vi "auton_parse.vi"() -> ()   [LabVIEW 2015]
doc: "This VI is called when autonomous begins, and will automatically be terminated when autonomous ends. You can carry out timed or sensor driven robot movement independently without needing to return to the caller."
uses:
  auto_data.vi
panel:
  in  "auton_names":string[](array[string])=["none.bee", "", "", "", "", ""]
  # "Read a list of files from the filesystem\nParse them all into a giant command vector array"
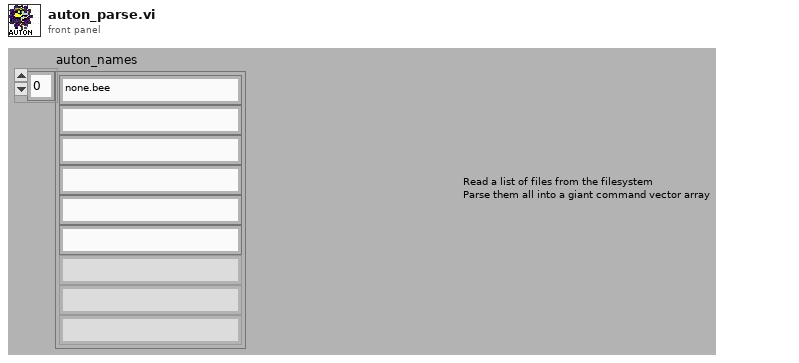
[diagram p1: front panel]
types:
  T1 = typedef "vi_execute.ctl" = cluster{"arguments":string[], "command":string, "refnum valid check":bool, "vi_ind":u8}
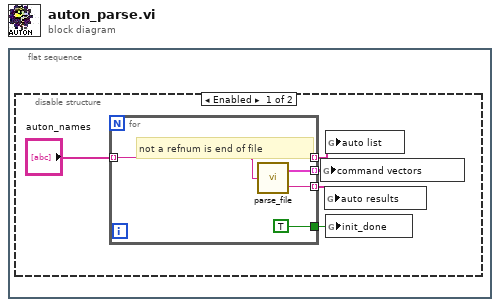
[diagram p0: block diagram]
diagram:
  n1 = flat-sequence {
    frame #0 {
      n2 = disable-structure shown="Enabled" {
        frame Enabled {
          n3 = for {
            tunnel: "auton_names" -> [w9] mode=indexing
            tunnel: [w9] -> w5 mode=indexing
            tunnel: [w6] -> w1 mode=indexing
            tunnel: [TRUE ("init_done")] -> w4
            tunnel: [w7] -> w2 mode=indexing
            # "not a refnum is end of file"
            n4 = call "parse_file.vi"("File Name With Extension"=w9) -> ("command vector"=w6:T1[], "file_status"=w7:string)
          }
          n5 = global write "auto_data.vi" "command vectors"(w1) -> ()
          n6 = global write "auto_data.vi" "auto results"(w2) -> ()
          n7 = global write "auto_data.vi" "auto list"(w5) -> ()
          n8 = global write "auto_data.vi" "init_done"(w4) -> ()
        }
        frame Disabled {
        }
      }
    }
  }
